vi "dgemv - General Matrix-Vector Product (DBL).vi"(4 "beta":dbl=1.0, 6 "alpha":dbl=1.0, 7 "operation A":T1 items=["Direct", "Conjugated & Transposed", "Transposed"], 9 "y":dbl[](array[numeric]), 10 "x":dbl[](array[numeric]), 11 "A":T2) -> (0 "error":i32, 3 "dgemv":dbl[](array[numeric]))   [LabVIEW 2020, in "NI_AALBLAS.lvlib"]
doc: "Calculates the product of a general matrix and a vector."
uses:
  NI_AALBLAS.lvlib
  RealMatrix.ctl
  LV_Transpose.ctl
  Fucntion.ctl
  Order.ctl
  NI_Matrix.lvlib
panel:
  # "dgemv=alpha*op(A)*x+beta*y"
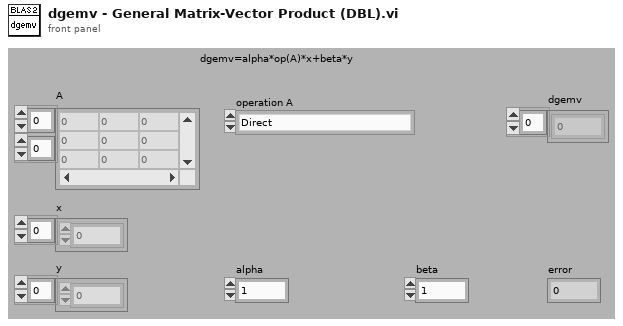
[diagram p1: front panel]
types:
  T1 = typedef "NI_AALBLAS.lvlib/LV_Transpose.ctl" = i32
  T2 = typedef "NI_Matrix.lvlib/RealMatrix.ctl" = dbl[][]
  T3 = typedef "NI_AALBLAS.lvlib/Order.ctl" = i32
  T4 = typedef "NI_AALBLAS.lvlib/Fucntion.ctl" = u16
  T5 = typedef "NI_AALBLAS.lvlib/Operation_Transpose.ctl" = i32
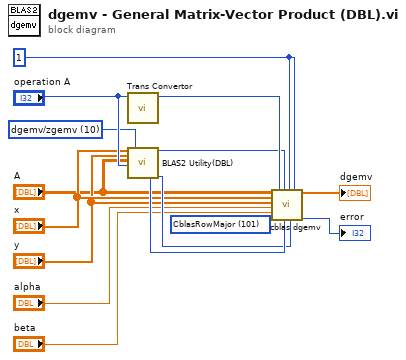
[diagram p0: block diagram]
diagram:
  w1 = 1
  w2 = T3 101 items=["CblasRowMajor"=101, "CblasColMajor"=102] ("order")
  w4 = T4 10 items=["ddot/zdotu/zdotc", "daxpy/zaxpy", "dnrm2/dznrm2", "dasum/dzasum", "dcopy/zcopy", "dswap/zswap", "drotm", "drot/zdrot", "idamax/izamax", "idamin/izamin", "dgemv/zgemv", "dsymv/zhemv", "dtrmv/ztrmv", "dsyr/zher", "dsyr2/zher2", "dger/zgeru/zgerc", "dtrsv/ztrsv", "dgemm/zgemm", "dsymm/zsymm/zhemm", "dtrmm/ztrmm", "dsyrk/zsyrk/zherk", "dsyr2k/zsyr2k/zher2k", "dtrsm/ztrsm"] ("function")
  n1 = call "Trans Convertor.vi"("operation"="operation A") -> ("trans"=w10:T5)  [unwired: 10 out]
  n2 = call "BLAS2 Utility(DBL).vi"("x"="x", "y"="y", "A"="A", "operation A"="operation A", "function"=w4) -> ("m"=w15:i32, "lda"=w3:i32, "n"=w14:i32)  [unwired: 12 in]
  n3 = call "cblas dgemv.vi"("A"="A", "x"="x", "y"="y", "alpha"="alpha", "beta"="beta", "order"=w2, "transA"=w10, "lda"=w3, "m"=w15, "incx"=w1, "n"=w14, "incy"=w1) -> ("dgemv"=→"dgemv":dbl[], "error"=→"error":i32)  [unwired: 6 out]
